vi "Tree Symbols-FG.vi"(7 "Actions":T1(ring), 8 "error in (no error)":errorcluster, 9 "Symbol Name":string, 10 "Item Tag":string, 11 "Tree Ref":refnum<vi>) -> (0 "error out":errorcluster, 1 "GlyphIndex":i32, 2 "Item Tag out":string, 3 "Tree Ref out":refnum<vi>)   [LabVIEW 2018]
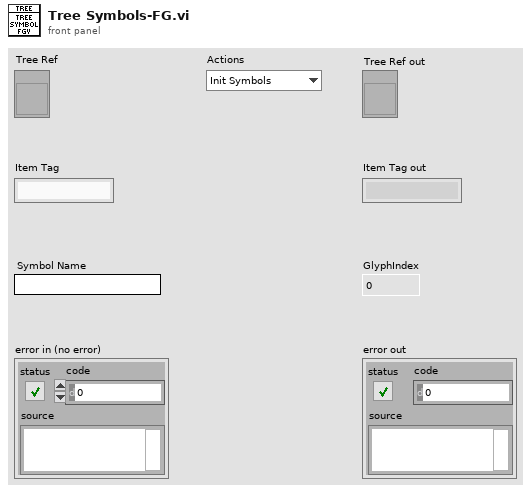
[diagram p1: front panel]
types:
  T1 = enum16{"Init Symbols", "Set Item Symbol", "Get Symbol Index"}
  T2 = typedef "imagedata.ctl" = cluster{"image type":i32, "image depth":i32, "image":u8[], "mask":u8[], "colors":u32[], "Rectangle":cluster{"left":i16, "top":i16, "right":i16, "bottom":i16}}
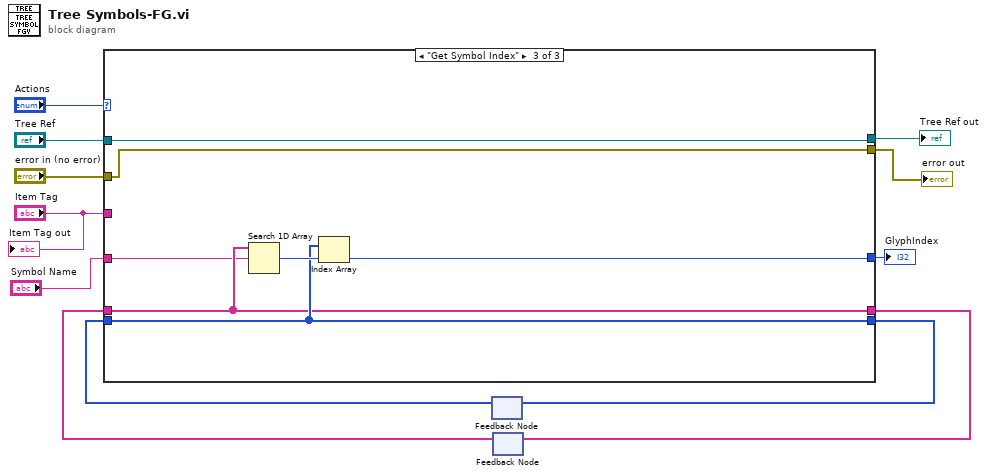
[diagram p0: block diagram]
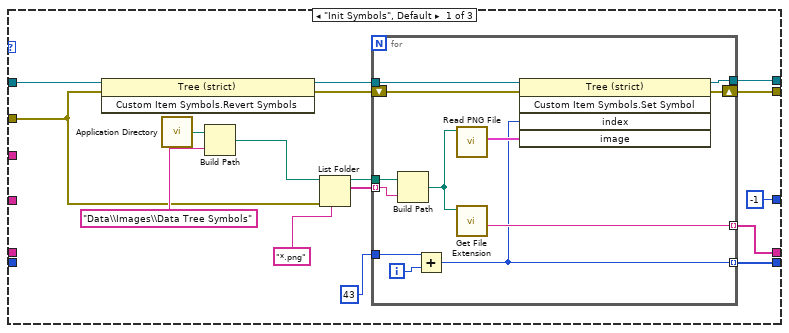
[diagram p2: hidden frame]
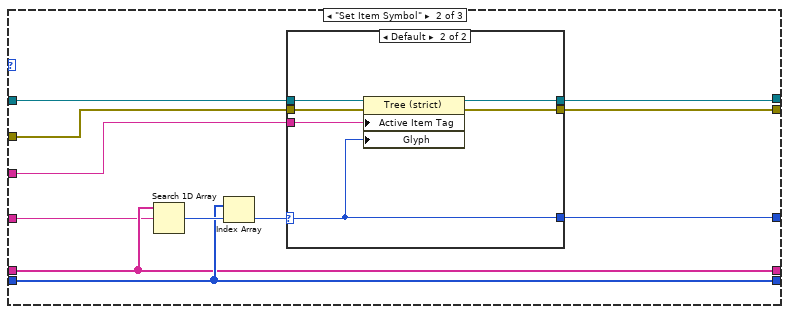
[diagram p3: hidden frame]
diagram:
  n1 = feedback #1() -> (w3:i32[])  [unwired: 1 in]
  n2 = feedback #2() -> (w4:string[])  [unwired: 1 in]
  n3 = case shown="\"Get Symbol Index\"" "Actions" {
    tunnel: "Tree Ref" -> [w28 w51 w67]
    tunnel: "error in (no error)" -> [w25 w50 w66]
    tunnel: [w17 w43 w62] -> w8
    tunnel: [w16 w44 w63] -> w9
    tunnel: [w15 w48 w67] -> w7
    tunnel: [w14 w47 w66] -> w6
    tunnel: "Item Tag" -> [_ w49 _]
    tunnel: w4 -> [_ w43 w62]
    tunnel: w3 -> [_ w44 w63]
    tunnel: [-1 ("index of element") w42 w64] -> w2
    tunnel: "Symbol Name" -> [_ w41 w61]
    frame "Init Symbols", Default {
      n4 = invoke class="Tree (strict)" method="Custom Item Symbols.Revert Symbols"(reference=w28, error in=w25) -> (reference out=w22:refnum<vi>, error out=w21:errorcluster)  [unwired: 1 in, 1 out]
      n5 = call <vilib>:"Application Directory.vi"() -> ("Application Directory"=w27:path)
      n6 = Build Path(base path=w27, name or relative path="Data\\Images\\Data Tree Symbols") -> (appended path=w24:path)
      n7 = List Folder(path=w24, pattern="*.png", error in=w25) -> (path out=w20:path, filenames=w19:string[])  [unwired: 1 in, 2 out]
      n8 = for {
        tunnel: w22 -> [w39]
        shift-right: [w40] -> w14
        shift-left: w21 -> [w38]
        tunnel: [w37] -> w15
        tunnel: w20 -> [w36]
        tunnel: w19 -> [w35] mode=indexing
        tunnel: [w32] -> w17 mode=indexing
        tunnel: 43 -> [w30]
        tunnel: [w29] -> w16 mode=indexing
        i -> [w31]
        n9 = Build Path(base path=w36, name or relative path=w35) -> (appended path=w33:path)
        n10 = Add(x=w30, y=w31) -> (x+y=w29:i32)
        n11 = call <vilib>:"Read PNG File.vi"("path to PNG file"=w33) -> ("image data"=w34:T2)  [unwired: 8 in, 2 out]
        n12 = call <vilib>:"Get File Extension.vi"("file"=w33) -> ("filename without extension"=w32:string)  [unwired: 6 in, 4 out]
        n13 = invoke class="Tree (strict)" method="Custom Item Symbols.Set Symbol"(reference=w39, error in=w38, "index"=w29, "image"=w34) -> (reference out=w37:refnum<vi>, error out=w40:errorcluster)  [unwired: 1 in, 3 out]
      }
    }
    frame "Set Item Symbol" {
      n14 = Search 1D Array(1D array=w43, element=w41) -> (index of element=w46:i32)  [unwired: 1 in]
      n15 = Index Array(array=w44, index=w46) -> (element=w45:i32)
      n16 = case shown="Default" w45 {
        selector: w45 -> [w52 w55]
        tunnel: w51 -> [w54 w60]
        tunnel: w50 -> [w53 w59]
        tunnel: w49 -> [_ w58]
        tunnel: [w54 w57] -> w48
        tunnel: [w53 w56] -> w47
        tunnel: [w52 w55] -> w42
        frame -1 {
        }
        frame Default {
          n17 = property class="Tree (strict)"(reference=w60, error in=w59, "Active Item Tag"=w58, "Glyph"=w55) -> (reference out=w57:refnum<vi>, error out=w56:errorcluster)
        }
      }
    }
    frame "Get Symbol Index" {
      n18 = Search 1D Array(1D array=w62, element=w61) -> (index of element=w65:i32)  [unwired: 1 in]
      n19 = Index Array(array=w63, index=w65) -> (element=w64:i32)
    }
  }
  "Tree Ref out" <- w7
  "error out" <- w6
  "GlyphIndex" <- w2
  n20 = feedback-in #1(w9) -> ()
  n21 = feedback-in #2(w8) -> ()
  "Item Tag out" <- "Item Tag"
